vi "Read_raw_inst_setup.vi"(0 "Setup file":string) -> (8 "Setup string":string, 10 "Ch & spans choices":T4[](array[typedef]) {"D" format="%.2f"; "Ch No" min=0; "low limit" min=-10 max=10 format="%.2f"; "high limit" min=-10 max=10 format="%.2f"}, 13 "PWA Data":T1, 14 "Number of Analogue instruments":i32=1, 16 "LDA data":enum16{"No LDA data", "Take LDA data"}(ring)=enum."Take LDA data", 17 "LDA set up":T3={"dimensions"=enum."2D", "Analogue Freq Multiplier"=0.1} {"Analogue Freq Multiplier" min=0.1 max=100.0 format="%_5g"}, 19 "Synchronise Analogue channels with LDA":bool)   [LabVIEW 2013]
uses:
  Controls/Ch_and_spans_choices.ctl
  Controls/Inst_type.ctl
  Controls/LDA_Setup.ctl
  Controls/PWA_Data.ctl
  Controls/Post_Process.ctl
  File/Setup_Filetype.ctl
  Controls/Trigger_Mode.ctl
  Controls/Tunnel_Coordinates.ctl
  Globals/Meas_global.vi
  Globals/LDA_meas_global_1.vi
  Globals/LDA_meas_global_2.vi
  Globals/Trav_pos_global.vi
panel:
  in  "Inst type":T2
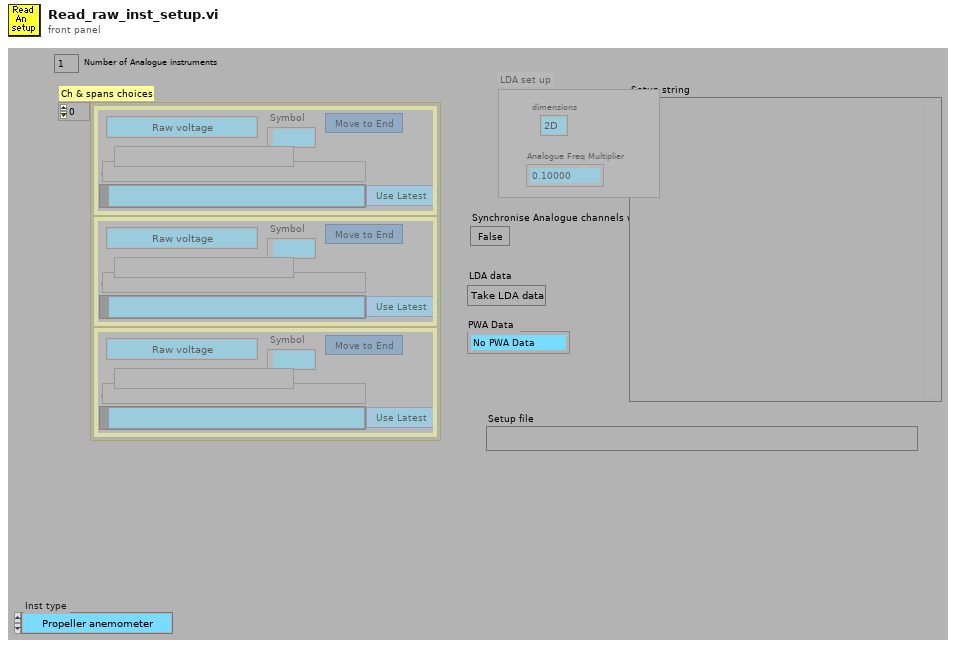
[diagram p1: front panel]
types:
  T1 = typedef "PWA_Data.ctl" = enum16{"No PWA Data", "One Ch PWA"}
  T2 = typedef "Inst_type.ctl" = enum16{"Propeller anemometer", "Raw voltage", "Pressure Transducer", "Pitot-static tube", "Preston tube", "Hot wire", "Cross wire 1", "Cross wire 2", "Generic Linear", "Generic Polynomial", "Generic BackPoly", "Fast FID", "Thermocouple", "Cold wire", "Pulsed Wire", "LDA Vel", "LDA Tran time", "LDA Arr time"}
  T3 = typedef "LDA_Setup.ctl" = cluster{"dimensions":enum16{"1D", "2D"}, "Analogue Freq Multiplier":dbl}
  T4 = typedef "Ch_and_spans_choices.ctl" = cluster{"high limit":sgl, "low limit":sgl, "Ch No":i16, "Calib filename":path, "Inst type":T2, "Symbol":string, "Move channel":bool, "Use Latest":bool, "D":dbl, "Ch Name":string, "DAQmx Physical Channel":tag}
  T5 = typedef "Post_Process.ctl" = enum16{"Take New Data", "Post Process Raw Data File"}
  T6 = typedef "Setup_Filetype.ctl" = enum16{"Measurement Setups", "Calibration Setups", "General", "Results File Plotter Setups", "Speed Calib Tweaks"}
  T7 = typedef "Trigger_Mode.ctl" = enum16{"Free Running", "Start on Trigger", "Trigger Every Block", "Trigger Every Sample"}
  T8 = typedef "Tunnel_Coordinates.ctl" = enum16{"Work in Tunnel Coordinates", "Work in Model Coordinates"}
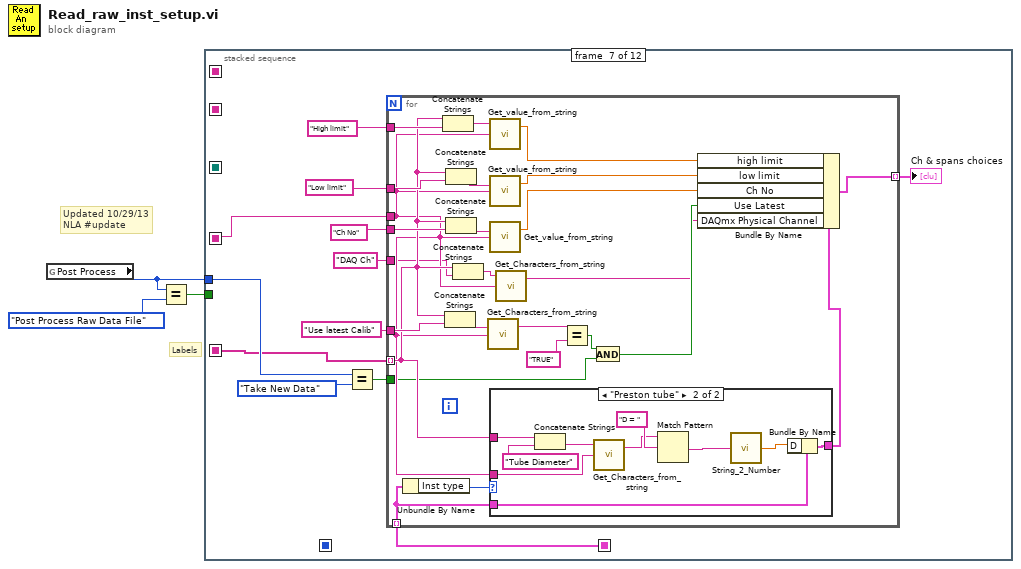
[diagram p0: block diagram]
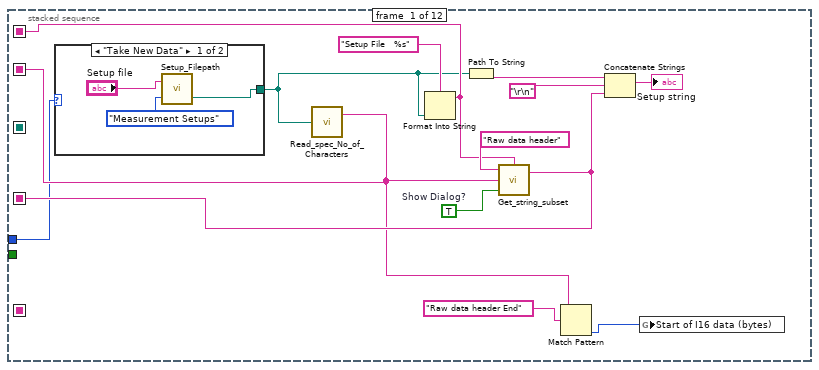
[diagram p2: hidden frame]
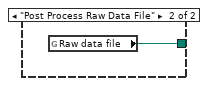
[diagram p3: hidden frame]
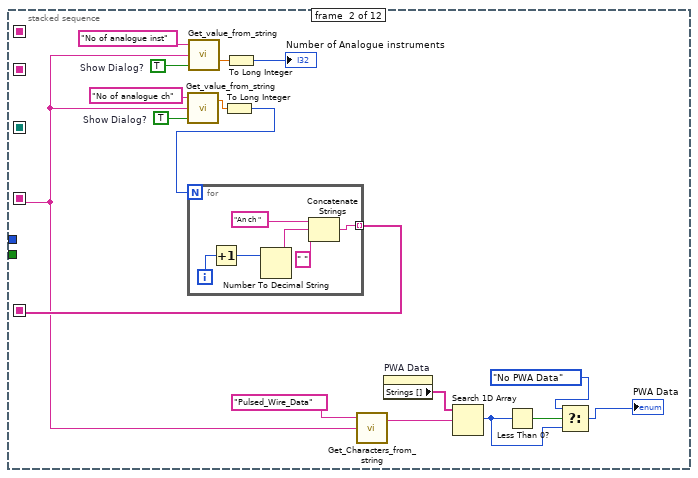
[diagram p4: hidden frame]
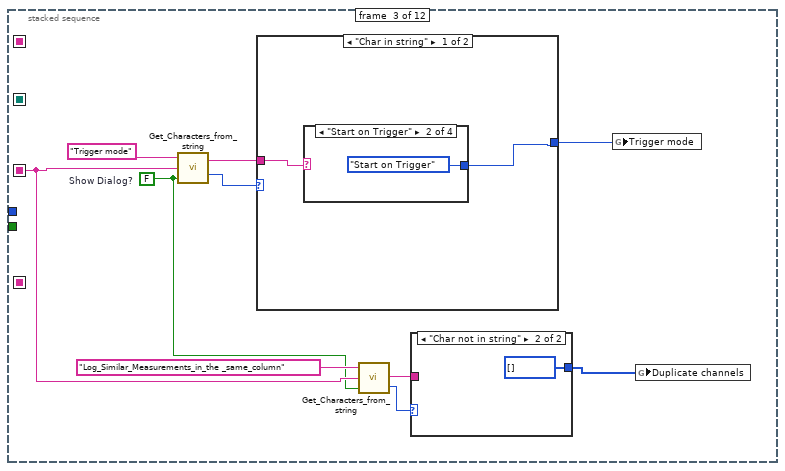
[diagram p5: hidden frame]
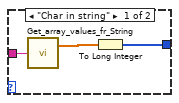
[diagram p6: hidden frame]
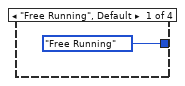
[diagram p7: hidden frame]
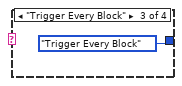
[diagram p8: hidden frame]
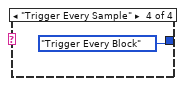
[diagram p9: hidden frame]
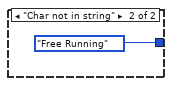
[diagram p10: hidden frame]
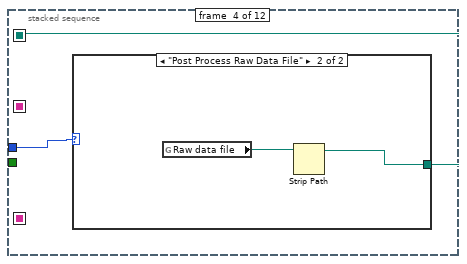
[diagram p11: hidden frame]
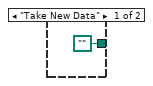
[diagram p12: hidden frame]
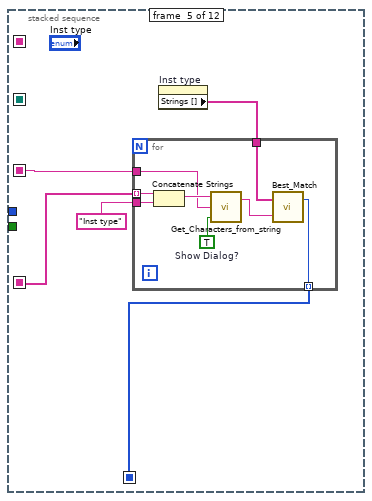
[diagram p13: hidden frame]
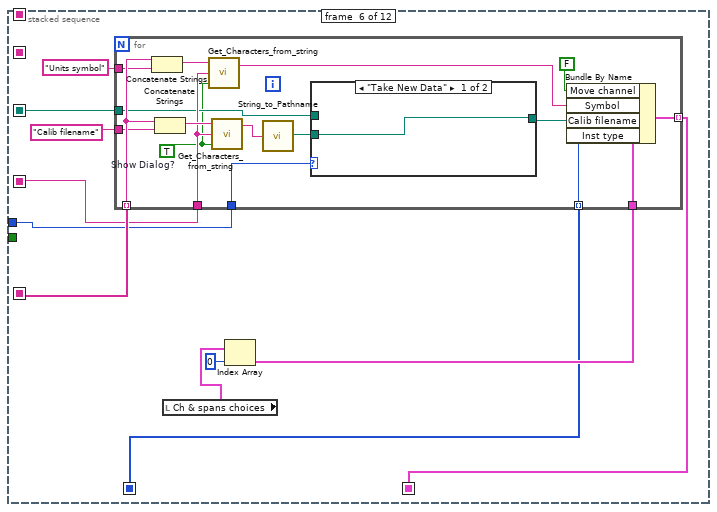
[diagram p14: hidden frame]
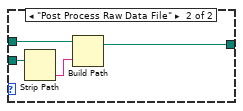
[diagram p15: hidden frame]
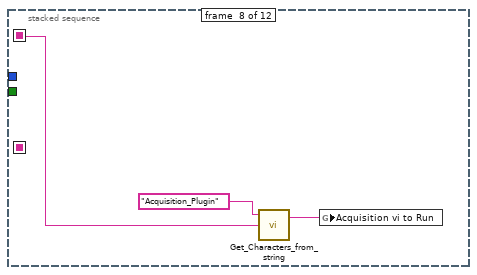
[diagram p17: hidden frame]
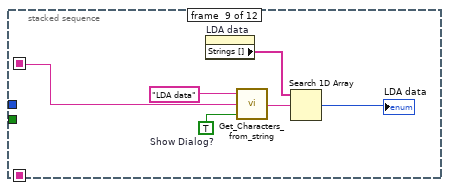
[diagram p18: hidden frame]
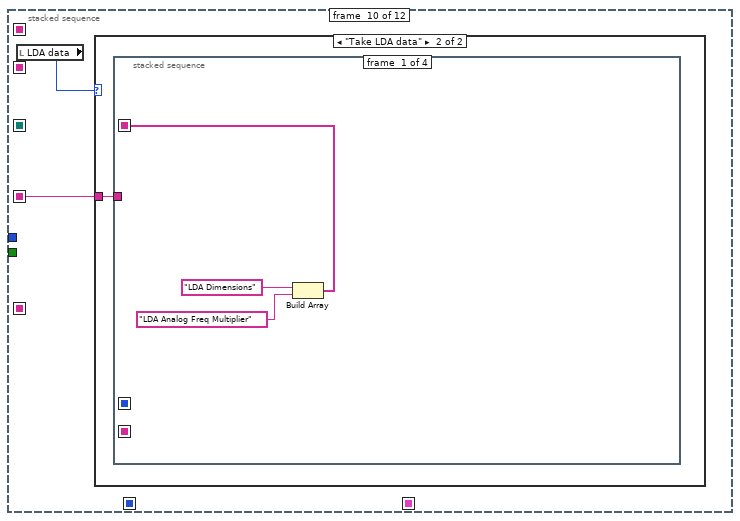
[diagram p19: hidden frame]
diagram:
  # "Updated 10/29/13\nNLA #update"
  # "Labels"
  n1 = global read "Meas_global.vi" "Post Process"() -> (w1:T5)
  n2 = Equal?(x=w1, y=Post_Process."Post Process Raw Data File" ("Post Process")) -> (x = y?=w3:bool)
  n3 = stacked-sequence {
    seq-local: [w14 _ _ _ _ _ _ _ _ _ _ _] -> [_ w28 w48 _ w74 w85 w127 w166 w171 w174 w236 w260]
    seq-local: [_ w35 _ _ _ _ _ _ _ _ _ _] -> [_ _ _ _ w73 w93 w119 _ _ _ _ _]
    seq-local: [_ _ _ _ w70 _ _ _ _ _ _ _] -> [_ _ _ _ _ w88 _ _ _ _ _ _]
    seq-local: [_ _ _ _ _ w87 _ _ _ _ _ _] -> [_ _ _ _ _ _ w126 _ _ _ _ _]
    seq-local: [_ _ _ w66 _ _ _ _ _ _ _ _] -> [_ _ _ _ _ w86 _ _ _ _ _ _]
    seq-local: [w9 _ _ _ _ _ _ _ _ _ _ _] -> [_ _ _ _ _ _ _ _ _ _ _ w259]
    seq-local: [w6 _ _ _ _ _ _ _ _ _ _ _] -> [_ _ _ _ _ _ _ _ _ _ _ _]
    tunnel: w3 -> [_ _ _ _ _ _ _ _ _ _ _ w261]
    tunnel: w1 -> [w5 _ _ w65 _ w84 w120 _ _ _ _ _]
    frame #0 {
      w11 = TRUE  # Show Dialog?
      n4 = case shown="\"Take New Data\"" w5 {
        tunnel: [w17 w20] -> w4
        frame "Take New Data" {
          n5 = call "Setup_Filepath.vi"("Setup File Type"=Setup_Filetype."Measurement Setups", "Filename in"="Setup file") -> ("Filename Out"=w17:path)  [unwired: 1 out]
        }
        frame "Post Process Raw Data File" {
          n6 = global read "Meas_global.vi" "Raw data file"() -> (w20:path)
        }
      }
      n7 = call "Read_spec_No_of_Characters.vi"("Filename"=w4) -> ("character string"=w9:string)  [unwired: 1 out]
      n8 = Format Into String(format string="Setup File   %s", w4) -> (resulting string=w6:string)  [unwired: 2 in, 1 out]
      n9 = Path To String(path=w4) -> (string=w12:string)
      n10 = call "Get_string_subset.vi"("String Name"=w6, "Show Dialog?"=w11, "String to split"=w9, "File Label"="Raw data header") -> ("Output string"=w14:string)  [unwired: 1 out]
      n11 = Match Pattern(string=w9, regular expression="Raw data header End") -> (offset past match=w8:i32)  [unwired: 4 out]
      n12 = Concatenate Strings(w12, "\r\n", w14) -> (→"Setup string":string)
      n13 = global write "Meas_global.vi" "Start of I16 data (bytes)"(w8) -> ()
    }
    frame #1 {
      w29 = TRUE  # Show Dialog?
      w30 = TRUE  # Show Dialog?
      n14 = call "Get_value_from_string.vi"("Show Dialog?"=w30, "Input string"=w28, "Variable name"="No of analogue ch") -> ("Value"=w36:dbl)  [unwired: 1 out]
      n15 = call "Get_value_from_string.vi"("Show Dialog?"=w29, "Input string"=w28, "Variable name"="No of analogue inst") -> ("Value"=w33:dbl)  [unwired: 1 out]
      n16 = To Long Integer(number=w36) -> (32bit integer=w31:i32)
      n17 = for {
        N: w31 -> [_]
        tunnel: [w39] -> w35 mode=indexing
        i -> [w41]
        n18 = Increment(x=w41) -> (x+1=w40:i32)
        n19 = Number To Decimal String(number=w40) -> (decimal integer string=w43:string)  [unwired: 1 out]
        n20 = Concatenate Strings("An ch ", w43, " ") -> (w39:string)
      }
      n21 = To Long Integer(number=w33) -> (32bit integer=→"Number of Analogue instruments":i32)
      n22 = call "Get_Characters_from_string.vi"("Input string"=w28, "Variable name"="Pulsed_Wire_Data") -> ("Value"=w25:string)  [unwired: 1 in, 1 out]
      n23 = property on="PWA Data" class="Enum (strict)"() -> ("Strings []"=w26:string[])  [unwired: 2 in, 2 out]
      n24 = Search 1D Array(1D array=w26, element=w25) -> (index of element=w22:i32)  [unwired: 1 out]
      n25 = Less Than 0?(x=w22) -> (x < 0?=w24:bool)
      n26 = Select(t=PWA_Data."No PWA Data" ("PWA Data"), s=w24, f=w22) -> (s? t:f=→"PWA Data":i32)
    }
    frame #2 {
      w47 = FALSE  # Show Dialog?
      n27 = call "Get_Characters_from_string.vi"("Show Dialog?"=w47, "Input string"=w48, "Variable name"="Trigger mode") -> ("Status"=w52:enum16{"Char in string", "Char not in string"}, "Value"=w51:string)
      n28 = case shown="\"Char in string\"" w52 {
        tunnel: [w58 Trigger_Mode."Free Running" ("Trigger mode")] -> w50
        tunnel: w51 -> [w59 _]
        frame "Char in string" {
          n29 = case shown="\"Start on Trigger\"" w59 {
            tunnel: [Trigger_Mode."Free Running" ("Trigger mode") Trigger_Mode."Start on Trigger" ("Trigger mode") Trigger_Mode."Trigger Every Block" ("Trigger mode") Trigger_Mode."Trigger Every Block" ("Trigger mode")] -> w58
            frame "Free Running", Default {
            }
            frame "Start on Trigger" {
            }
            frame "Trigger Every Block" {
            }
            frame "Trigger Every Sample" {
            }
          }
        }
        frame "Char not in string" {
        }
      }
      n30 = call "Get_Characters_from_string.vi"("Show Dialog?"=w47, "Input string"=w48, "Variable name"="Log_Similar_Measurements_in_the _same_column") -> ("Status"=w44:enum16{"Char in string", "Char not in string"}, "Value"=w46:string)
      n31 = case shown="\"Char not in string\"" w44 {
        tunnel: w46 -> [w56 _]
        tunnel: [w54 i32[] []] -> w45
        frame "Char in string" {
          n32 = call "Get_array_values_fr_String.vi"("String Value"=w56) -> ("Numeric Array"=w55:dbl[])  [unwired: 1 out]
          n33 = To Long Integer(number=w55) -> (32bit integer=w54:i32[])
        }
        frame "Char not in string" {
        }
      }
      n34 = global write "Meas_global.vi" "Trigger mode"(w50) -> ()
      n35 = global write "Meas_global.vi" "Duplicate channels"(w45) -> ()
    }
    frame #3 {
      n36 = case shown="\"Post Process Raw Data File\"" w65 {
        tunnel: [path "" ("stripped path") w68] -> w66
        frame "Take New Data" {
        }
        frame "Post Process Raw Data File" {
          n37 = global read "Meas_global.vi" "Raw data file"() -> (w69:path)
          n38 = Strip Path(path=w69) -> (stripped path=w68:path)  [unwired: 1 out]
        }
      }
    }
    frame #4 {
      n39 = property on="Inst type" class="Enum (strict)"() -> ("Strings []"=w71:string[])  [unwired: 2 in, 2 out]
      n40 = for {
        tunnel: w74 -> [w81]
        tunnel: w71 -> [w77]
        tunnel: w73 -> [w80] mode=indexing
        tunnel: "Inst type" -> [w79]
        tunnel: [w75] -> w70 mode=indexing
        w78 = TRUE  # Show Dialog?
        n41 = Concatenate Strings(w80, w79) -> (w82:string)
        n42 = call "Get_Characters_from_string.vi"("Show Dialog?"=w78, "Input string"=w81, "Variable name"=w82) -> ("Value"=w76:string)  [unwired: 1 out]
        n43 = call "Best_Match.vi"("Input String"=w76, "String Options"=w77) -> ("index of element"=w75:i32)  [unwired: 1 out]
      }
    }
    frame #5 {
      n44 = local read "Ch & spans choices"() -> (w83:T4[])
      n45 = Index Array(array=w83, index=0) -> (element=w89:T4)
      n46 = for {
        tunnel: w93 -> [w108] mode=indexing
        tunnel: "Calib filename" -> [w107]
        tunnel: "Units symbol" -> [w106]
        tunnel: w89 -> [w105]
        tunnel: w88 -> [w103] mode=indexing
        tunnel: [w102] -> w87 mode=indexing
        tunnel: w85 -> [w101]
        tunnel: w84 -> [w100]
        tunnel: w86 -> [w99]
        w96 = TRUE  # Show Dialog?
        n47 = Concatenate Strings(w108, w106) -> (w110:string)
        n48 = Concatenate Strings(w108, w107) -> (w109:string)
        n49 = call "Get_Characters_from_string.vi"("Show Dialog?"=w96, "Input string"=w101, "Variable name"=w110) -> ("Value"=w104:string)  [unwired: 1 out]
        n50 = call "Get_Characters_from_string.vi"("Show Dialog?"=w96, "Input string"=w101, "Variable name"=w109) -> ("Value"=w95:string)  [unwired: 1 out]
        n51 = call "String_to_Pathname.vi"("Input String"=w95) -> ("path"=w94:path)
        n52 = case shown="\"Take New Data\"" w100 {
          tunnel: w94 -> [w111 w115]
          tunnel: w99 -> [_ w112]
          tunnel: [w111 w113] -> w98
          frame "Take New Data" {
          }
          frame "Post Process Raw Data File" {
            n53 = Strip Path(path=w115) -> (name=w114:string)  [unwired: 1 out]
            n54 = Build Path(base path=w112, name or relative path=w114) -> (appended path=w113:path)
          }
        }
        n55 = Bundle By Name(cluster=w105, "Move channel"=FALSE, "Symbol"=w104, "Calib filename"=w98, "Inst type"=w103) -> (w102:T4)
      }
    }
    frame #6 {
      n56 = Equal?(x=w120, y=Post_Process."Take New Data" ("Post Process")) -> (x = y?=w118:bool)
      n57 = for {
        tunnel: "Low limit" -> [w152]
        tunnel: "High limit" -> [w151]
        tunnel: w126 -> [w137] mode=indexing
        tunnel: [w135] -> w116 mode=indexing
        tunnel: w127 -> [w139]
        tunnel: "Ch No" -> [w147]
        tunnel: "Use latest Calib" -> [w145]
        tunnel: w119 -> [w140] mode=indexing
        tunnel: w118 -> [w138]
        tunnel: "DAQ Ch" -> [w130]
        n58 = Unbundle By Name(w137) -> ("Inst type"=w141:T2)
        n59 = Concatenate Strings(w140, w151) -> (w150:string)
        n60 = Concatenate Strings(w140, w145) -> (w146:string)
        n61 = Concatenate Strings(w140, w152) -> (w149:string)
        n62 = Concatenate Strings(w140, w147) -> (w148:string)
        n63 = Concatenate Strings(w140, w130) -> (w131:string)
        n64 = call "Get_Characters_from_string.vi"("Input string"=w139, "Variable name"=w146) -> ("Value"=w144:string)  [unwired: 1 in, 1 out]
        n65 = call "Get_value_from_string.vi"("Input string"=w139, "Variable name"=w150) -> ("Value"=w129:dbl)  [unwired: 1 in, 1 out]
        n66 = call "Get_value_from_string.vi"("Input string"=w139, "Variable name"=w149) -> ("Value"=w133:dbl)  [unwired: 1 in, 1 out]
        n67 = call "Get_value_from_string.vi"("Input string"=w139, "Variable name"=w148) -> ("Value"=w128:dbl)  [unwired: 1 in, 1 out]
        n68 = case shown="\"Preston tube\"" w141 {
          tunnel: w140 -> [_ w163]
          tunnel: w139 -> [_ w158]
          tunnel: w137 -> [w153 w161]
          tunnel: [w153 w160] -> w136
          frame "Propeller anemometer", Default {
          }
          frame "Preston tube" {
            n69 = Concatenate Strings(w163, "Tube Diameter") -> (w159:string)
            n70 = call "Get_Characters_from_string.vi"("Input string"=w158, "Variable name"=w159) -> ("Value"=w156:string)  [unwired: 1 in, 1 out]
            n71 = Match Pattern(string=w156, regular expression="D = " ("String to match")) -> (after substring=w155:string)  [unwired: 4 out]
            n72 = call "String_2_Number.vi"("Value"=w155) -> ("Numeric"=w154:dbl)
            n73 = Bundle By Name(cluster=w161, "D"=w154) -> (w160:T4)
          }
        }
        n74 = call "Get_Characters_from_string.vi"("Input string"=w139, "Variable name"=w131) -> ("Value"=w132:string)  [unwired: 1 in, 1 out]
        n75 = Equal?(x=w144, y="TRUE") -> (x = y?=w142:bool)
        n76 = And(x=w142, y=w138) -> (x .and. y?=w134:bool)
        n77 = Bundle By Name(cluster=w136, "high limit"=w129, "low limit"=w133, "Ch No"=w128, "Use Latest"=w134, "DAQmx Physical Channel"=w132) -> (w135:T4)
      }
      "Ch & spans choices" <- w116
    }
    frame #7 {
      n78 = call "Get_Characters_from_string.vi"("Input string"=w166, "Variable name"="Acquisition_Plugin") -> ("Value"=w164:string)  [unwired: 1 in, 1 out]
      n79 = global write "Meas_global.vi" "Acquisition vi to Run"(w164) -> ()
    }
    frame #8 {
      w168 = TRUE  # Show Dialog?
      n80 = property on="LDA data" class="Enum (strict)"() -> ("Strings []"=w167:string[])  [unwired: 2 in, 2 out]
      n81 = call "Get_Characters_from_string.vi"("Show Dialog?"=w168, "Input string"=w171, "Variable name"="LDA data" ("Label for characters")) -> ("Value"=w172:string)  [unwired: 1 out]
      n82 = Search 1D Array(1D array=w167, element=w172) -> (index of element=→"LDA data":i32)  [unwired: 1 out]
    }
    frame #9 {
      n83 = local read "LDA data"() -> (w173:enum16{"No LDA data", "Take LDA data"})
      n84 = case shown="\"Take LDA data\"" w173 {
        tunnel: w174 -> [_ w175]
        frame "No LDA data" {
        }
        frame "Take LDA data" {
          n85 = stacked-sequence {
            seq-local: [_ w181 _ _] -> [_ _ w207 _]
            seq-local: [_ _ w206 _] -> [_ _ _ w217]
            seq-local: [w177 _ _ _] -> [_ w183 _ _]
            tunnel: w175 -> [_ w180 _ w218]
            frame #0 {
              n86 = Build Array("LDA Dimensions", "LDA Analog Freq Multiplier") -> (w177:string[])
            }
            frame #1 {
              n87 = local read "LDA set up"() -> (w182:T3)
              n88 = for {
                tunnel: w183 -> [w189] mode=indexing
                shift-right: [w186] -> w179
                shift-left: w182 -> [w187]
                tunnel: w180 -> [w184]
                n89 = call "Get_Characters_from_string.vi"("Input string"=w184, "Variable name"=w189) -> ("Status"=w188:enum16{"Char in string", "Char not in string"}, "Value"=w185:string)  [unwired: 1 in]
                n90 = case shown="\"Char in string\"" w188 {
                  tunnel: w189 -> [w193 _]
                  tunnel: w187 -> [w192 w205]
                  tunnel: [w191 w205] -> w186
                  tunnel: w185 -> [w190 _]
                  frame "Char in string" {
                    n91 = case shown="\"LDA Analog Freq Multiplier\"" w193 {
                      tunnel: w192 -> [w197 w203 w204]
                      tunnel: [w196 w202 w204] -> w191
                      tunnel: w190 -> [w195 w201 _]
                      frame "LDA Dimensions" {
                        n92 = case shown="\"2D\", Default" w195 {
                          tunnel: [enum16{"1D", "2D"}."1D" ("Bundle Element") enum16{"1D", "2D"}."2D" ("Bundle Element")] -> w194
                          frame "1D" {
                          }
                          frame "2D", Default {
                          }
                        }
                        n93 = Bundle By Name(cluster=w197, "dimensions"=w194) -> (w196:T3)
                      }
                      frame "LDA Analog Freq Multiplier" {
                        n94 = Fract/Exp String To Number(string=w201) -> (number=w200:dbl)  [unwired: 3 in, 1 out]
                        n95 = Bundle By Name(cluster=w203, "Analogue Freq Multiplier"=w200) -> (w202:T3)
                      }
                      frame "No Match", Default {
                      }
                    }
                  }
                  frame "Char not in string" {
                  }
                }
              }
              "LDA set up" <- w179
              n96 = Unbundle By Name(w179) -> ("dimensions"=w181:enum16{"1D", "2D"})
            }
            frame #2 {
              n97 = case shown="\"1D\"" w207 {
                tunnel: [1 2] -> w208
                frame "1D" {
                }
                frame "2D" {
                }
              }
              n98 = for {
                N: w208 -> [_]
                tunnel: [w210] -> w206 mode=indexing
                i -> [w212]
                n99 = Increment(x=w212) -> (x+1=w211:i32)
                n100 = Number To Decimal String(number=w211) -> (decimal integer string=w214:string)  [unwired: 1 out]
                n101 = Concatenate Strings("BSA ", w214, " ") -> (w210:string)
              }
            }
            frame #3 {
              n102 = for {
                tunnel: w218 -> [w220]
                tunnel: w217 -> [w221] mode=indexing
                i -> [w230]
                n103 = Concatenate Strings(w221, "Component") -> (w231:string)
                n104 = Concatenate Strings(w221, "Multiply Velocity by -1") -> (w225:string)
                n105 = Increment(x=w230) -> (x+1=w227:i32)
                n106 = call "Get_Characters_from_string.vi"("Input string"=w220, "Variable name"=w231) -> ("Value"=w228:string)  [unwired: 1 in, 1 out]
                n107 = call "Get_Characters_from_string.vi"("Show Dialog?"=FALSE, "Input string"=w220, "Variable name"=w225) -> ("Value"=w223:string)  [unwired: 1 out]
                n108 = Equal?(x=w223, y="TRUE") -> (x = y?=w219:bool)
                n109 = case shown="2" w227 {
                  tunnel: w228 -> [w233 w235]
                  tunnel: w219 -> [w232 w234]
                  frame 1, Default {
                    n110 = global write "LDA_meas_global_1.vi" "Vel Comp BSA1"(w233) -> ()
                    n111 = global write "LDA_meas_global_1.vi" "Multiply Velocity by -1"(w232) -> ()
                  }
                  frame 2 {
                    n112 = global write "LDA_meas_global_2.vi" "Vel Comp BSA2"(w235) -> ()
                    n113 = global write "LDA_meas_global_2.vi" "Multiply Velocity by -1"(w234) -> ()
                  }
                }
              }
            }
          }
        }
      }
    }
    frame #10 {
      n114 = Build Array("Synchronise with LDA") -> (w246:string[])
      n115 = Build Array("FALSE", "TRUE") -> (w243:string[])
      n116 = call "Get_value_from_string.vi"("Input string"=w236, "Variable name"="Sync Delay Time (ms)" ("Label for characters")) -> ("Status"=w238:enum16{"Char in string", "Char not in string"}, "Value"=w237:dbl)  [unwired: 1 in]
      n117 = case shown="\"Char in string\"" w238 {
        tunnel: w237 -> [w248 _]
        frame "Char in string" {
          n118 = global write "LDA_meas_global_1.vi" "Sync Delay Time (ms)"(w248) -> ()
        }
        frame "Char not in string" {
        }
      }
      n119 = Build Array(FALSE, TRUE) -> (w240:bool[])
      n120 = for {
        tunnel: w236 -> [w256]
        tunnel: w246 -> [w252] mode=indexing
        tunnel: w243 -> [w251]
        tunnel: w240 -> [w250]
        i -> [w254]
        w249 = TRUE  # Show Dialog?
        n121 = call "Get_Characters_from_string.vi"("Show Dialog?"=w249, "Input string"=w256, "Variable name"=w252) -> ("Value"=w257:string)  [unwired: 1 out]
        n122 = Search 1D Array(1D array=w251, element=w257) -> (index of element=w255:i32)  [unwired: 1 out]
        n123 = Index Array(array=w250, index=w255) -> (element=w253:bool)
        n124 = case shown="1" w254 {
          tunnel: w253 -> [w258 _]
          frame 0, Default {
            "Synchronise Analogue channels with LDA" <- w258
          }
          frame 1 {
          }
        }
      }
    }
    frame #11 {
      n125 = case shown="True" w261 {
        tunnel: w260 -> [_ w267]
        tunnel: w259 -> [_ w262]
        frame False {
        }
        frame True {
          w266 = FALSE  # Show Dialog?
          n126 = call "Get_Characters_from_string.vi"("Show Dialog?"=w266, "Input string"=w267, "Variable name"="Coordinate_System" ("Label for characters")) -> ("Status"=w265:enum16{"Char in string", "Char not in string"}, "Value"=w264:string)
          n127 = case shown="\"Char not in string\"" w265 {
            tunnel: w264 -> [w270 _]
            tunnel: [w269 w273] -> w263
            tunnel: w262 -> [_ w275]
            frame "Char in string" {
              n128 = case shown="\"Work in Model Coordinates\"" w270 {
                tunnel: [Tunnel_Coordinates."Work in Model Coordinates" ("Work in Tunnel Coordinates?") Tunnel_Coordinates."Work in Tunnel Coordinates" ("Work in Tunnel Coordinates?")] -> w269
                frame "Work in Model Coordinates" {
                }
                frame "Work in Tunnel Coordinates", Default {
                }
              }
            }
            frame "Char not in string" {
              n129 = Concatenate Strings("X Pos (Model)", "\t", "Y Pos (Model)") -> (w276:string)
              n130 = Match Pattern(string=w275, regular expression=w276) -> (offset past match=w274:i32)  [unwired: 4 out]
              n131 = case shown="-1" w274 {
                tunnel: [Tunnel_Coordinates."Work in Model Coordinates" ("Work in Tunnel Coordinates?") Tunnel_Coordinates."Work in Tunnel Coordinates" ("Work in Tunnel Coordinates?")] -> w273
                frame 0, Default {
                }
                frame -1 {
                }
              }
            }
          }
          n132 = global write "Trav_pos_global.vi" "Work in Tunnel Coordinates?"(w263) -> ()
        }
      }
    }
  }
